vi "minxy.vi"(10 "y":dbl, 11 "x in":dbl) -> (3 "x out":dbl)   [LabVIEW 2014]
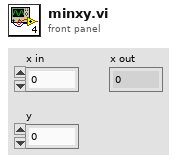
[diagram p1: front panel]
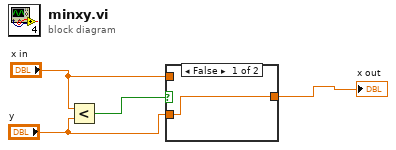
[diagram p0: block diagram]
diagram:
  n1 = Less?(x="x in", y="y") -> (x < y?=w1:bool)
  n2 = case shown="False" w1 {
    tunnel: "y" -> [w5 _]
    tunnel: "x in" -> [_ w6]
    tunnel: [w5 w6] -> w4
    frame False {
    }
    frame True {
    }
  }
  "x out" <- w4
